vi "Calc_Scale Value.vi"(0 "Normalized Value":dbl, 7 "Max":dbl, 9 "Min":dbl) -> (14 "Value":dbl)   [LabVIEW 2017]
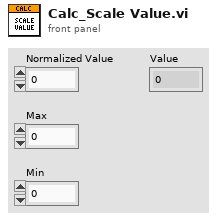
[diagram p1: front panel]
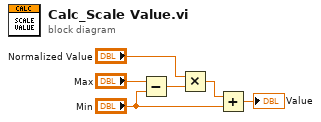
[diagram p0: block diagram]
diagram:
  n1 = Subtract(x="Max", y="Min") -> (x-y=w4:dbl)
  n2 = Multiply(x="Normalized Value", y=w4) -> (x*y=w1:dbl)
  n3 = Add(x=w1, y="Min") -> (x+y=→"Value":dbl)
